vi "Update User Interface.vi"(8 "error in (no error)":errorcluster, 10 "Refnum":refnum<vi>, 11 "Sequencer in":refnum<class "Sequencer.lvclass">) -> (0 "error out":errorcluster, 3 "Sequencer out":refnum<class "Sequencer.lvclass">)   [LabVIEW 2024, in "Ramses Sequencer.lvlib" / "Sequencer.lvclass"]
uses:
  Sequencer.lvclass
  Base Step/Base Step.lvclass/Base Step.ctl
  <vilib>/Utility/miscctls.llb/LVRowAndColumnTypeDef.ctl
  Sequence/Sequence.lvclass
  Base Step/Base Step.lvclass
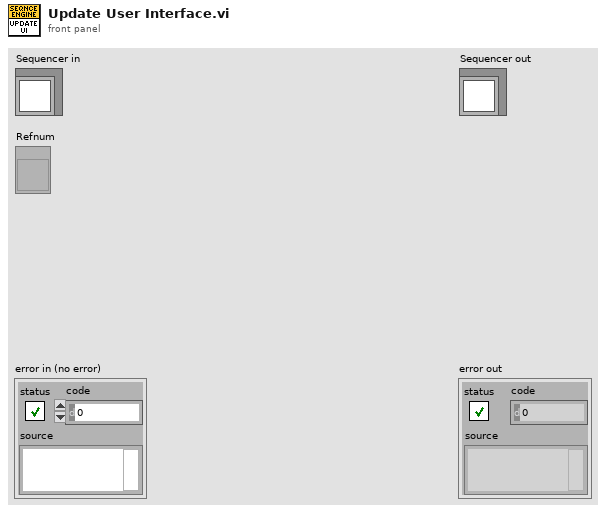
[diagram p1: front panel]
types:
  T1 = typedef "LVRowAndColumnTypeDef.ctl" = cluster{"Row":i32, "Column":i32}
  T2 = typedef "Ramses Sequencer.lvlib/Base Step.lvclass/Step State.ctl" = cluster{"Result":string, "Status":string, "Enabled":bool, "Upper":string, "Target":string, "Lower":string, "Value":string}
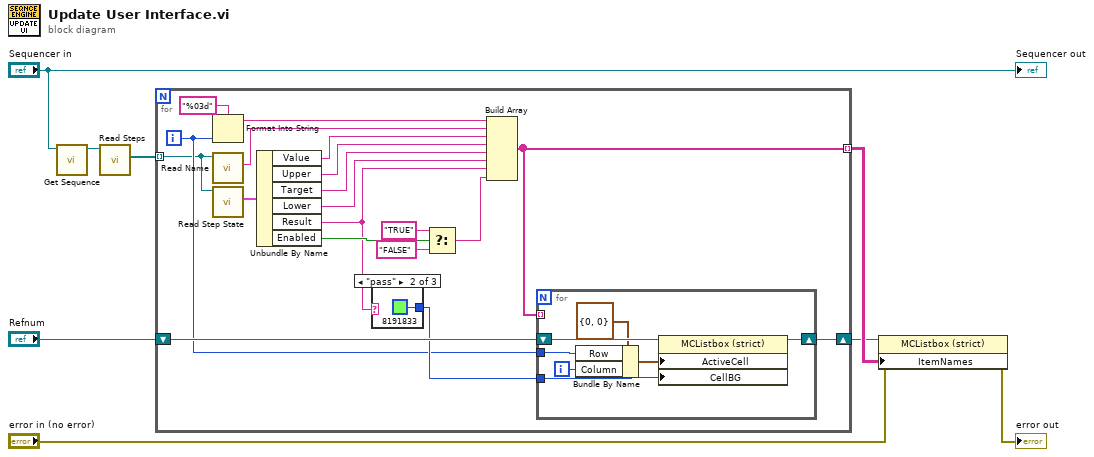
[diagram p0: block diagram]
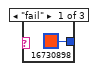
[diagram p2: hidden frame]
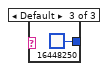
[diagram p3: hidden frame]
diagram:
  n1 = call "Get Sequence.vi"("Sequencer in"="Sequencer in") -> ("Sequence"=w8:refnum<class "Sequence.lvclass">)  [unwired: 9 in, 1 out]
  n2 = call-dynamic "Read Steps.vi"("Sequence in"=w8) -> ("Steps"=w7:refnum<class "Base Step.lvclass">[])  [unwired: 8 in, 2 out]
  n3 = for {
    tunnel: w7 -> [w10] mode=indexing
    tunnel: [w12] -> w3 mode=indexing
    shift-right: [w14] -> w1
    shift-left: "Refnum" -> [w15]
    i -> [w11]
    n4 = Format Into String(format string="%03d", w11) -> (resulting string=w26:string)  [unwired: 2 in, 1 out]
    n5 = call-dynamic "Read Name.vi"("Base Step in"=w10) -> ("Name"=w25:string)  [unwired: 8 in, 2 out]
    n6 = call "Read Step State.vi"("Base Step in"=w10) -> ("Step State"=w9:T2)  [unwired: 8 in, 2 out]
    n7 = Unbundle By Name(w9) -> ("Value"=w24:string, "Upper"=w23:string, "Target"=w22:string, "Lower"=w21:string, "Result"=w16:string, "Enabled"=w19:bool)
    n8 = case shown="\"pass\"" w16 {
      tunnel: [u32 16730898 ("Color") u32 8191833 ("Color") u32 16448250 ("Color")] -> w13
      frame "fail" {
      }
      frame "pass" {
      }
      frame Default {
      }
    }
    n9 = Select(t="TRUE" ("format string"), s=w19, f="FALSE" ("format string")) -> (s? t:f=w17:string)
    n10 = Build Array(w26, w25, w24, w23, w22, w21, w16, w17) -> (w12:string[])
    n11 = for {
      tunnel: w13 -> [w32]
      shift-right: [w33] -> w14
      shift-left: w15 -> [w34]
      tunnel: w12 -> [_] mode=indexing
      tunnel: w11 -> [w29]
      i -> [w28]
      n12 = Bundle By Name(cluster=T1 {"Row"=0, "Column"=0} ("Active Cell:Active Cell"), "Row"=w29, "Column"=w28) -> (w30:T1)
      n13 = property class="MCListbox (strict)"(reference=w34, "ActiveCell"=w30, "CellBG"=w32) -> (reference out=w33:refnum<vi>)  [unwired: 1 in, 1 out]
    }
  }
  n14 = property class="MCListbox (strict)"(reference=w1, error in="error in (no error)", "ItemNames"=w3) -> (error out=→"error out":errorcluster)  [unwired: 1 out]
  "Sequencer out" <- "Sequencer in"
